vi "参数配置.vi"() -> ()   [LabVIEW 2012]
doc: "打开板卡操作，输出板卡句柄！当有多个板卡时，根据板卡索引号打开不同板卡！\n如果同时使用一块板卡的多种功能，可将输出句柄连接到不同的功能任务中。\n此VI是创建所有任务的前提！"
panel:
  in  "50_100HZ 2":u32(ring) items=["50Hz脉冲", "100Hz脉冲"]
  in  "50_100HZ":u32(ring) items=["50Hz脉冲", "100Hz脉冲"]
  in  "马尔科夫脉冲强度 2":u32(ring) items=["0dB", "3dB", "6dB", "9dB", "12dB", "15dB", "18dB"]
  in  "马尔科夫种类 2":u32(ring) items=["弱马尔科夫", "中马尔科夫", "强马尔科夫"]
  in  "脉冲噪声开关 2":bool=TRUE
  in  "工频异步脉冲强度 2":u32(ring) items=["0dB", "3dB", "6dB", "9dB", "12dB", "15dB", "18dB"]
  in  "脉冲种类 2":u32(ring) items=["50KHz脉冲", "100KHz脉冲", "200KHz脉冲"]
  in  "工频异步噪声开关 2":bool=TRUE
  in  "周期噪声强度 2":u32(ring) items=["0dB", "3dB", "6dB", "9dB", "12dB", "15dB", "18dB"]
  in  "工频同步噪声开关 2":bool=TRUE
  in  "窄带噪声强度 2":u32(ring) items=["0dB", "3dB", "6dB", "9dB", "12dB", "15dB"]
  in  "11MHz 2":bool
  in  "7MHz 2":bool
  in  "3MHz 2":bool=TRUE
  in  "窄带噪声开关 2":bool=TRUE
  in  "白噪声色噪声切换 2":bool=TRUE
  in  "背景噪声开关 2":bool=TRUE
  in  "背景噪声强度 2":u32(ring) items=["0dB", "3dB", "6dB", "9dB", "12dB", "15dB", "18dB"]
  out "Points to Date 3":u32 caption="当前点数"
  out "Number Unread 3":i32 caption="未读取数字"
  out "Buffer Size 3":i32 caption="缓冲区大小"
  in  "马尔科夫脉冲强度":u32(ring) items=["0dB", "3dB", "6dB", "9dB", "12dB", "15dB", "18dB"]
  in  "马尔科夫种类":u32(ring) items=["弱马尔科夫", "中马尔科夫", "强马尔科夫"]
  in  "脉冲噪声开关":bool=TRUE
  in  "工频异步脉冲强度":u32(ring) items=["0dB", "3dB", "6dB", "9dB", "12dB", "15dB", "18dB"]
  in  "脉冲种类":u32(ring) items=["50KHz脉冲", "100KHz脉冲", "200KHz脉冲"]
  in  "工频异步噪声开关":bool=TRUE
  in  "周期噪声强度":u32(ring) items=["0dB", "3dB", "6dB", "9dB", "12dB", "15dB", "18dB"]
  in  "工频同步噪声开关":bool=TRUE
  in  "窄带噪声强度":u32(ring) items=["0dB", "3dB", "6dB", "9dB", "12dB", "15dB"]
  in  "11MHz":bool
  in  "7MHz":bool
  in  "3MHz":bool=TRUE
  in  "窄带噪声开关":bool=TRUE
  in  "白噪声色噪声切换":bool=TRUE
  in  "背景噪声开关":bool=TRUE
  in  "背景噪声强度":u32(ring) items=["0dB", "3dB", "6dB", "9dB", "12dB", "15dB", "18dB"]
  in  "取消按钮":bool
  in  "后向信道参数选择":u16(ring)=1 items=["禁用信道", "接入参考信道  类型1", "接入参考信道  类型2", "接入参考信道  类型3", "接入参考信道  类型4", "接入参考信道  类型5", "室内信道 类型1", "室内信道 类型2", "室内信道 类型3", "室内信道 类型4", "来自配置文件"]
  in  "布尔 4":bool
  in  "后项配置文件路径":path
  in  "前向信道参数选择":u16(ring)=6 items=["禁用信道", "接入参考信道  类型1", "接入参考信道  类型2", "接入参考信道  类型3", "接入参考信道  类型4", "接入参考信道  类型5", "室内信道  类型1", "室内信道  类型2", "室内信道  类型3", "室内信道  类型4", "来自配置文件"]
  in  "布尔 3":bool
  in  "前向配置文件路径":path
  out "Points to Date":u32 caption="当前点数"
  out "Number Unread":i32 caption="未读取数字"
  out "Buffer Size":i32 caption="缓冲区大小"
  in  "确定按钮":bool
  # "按下“绘制”按钮时，通过打开的子VI显示最近获取的1024个数据点，然后进行绘制。"
  # "背景噪声"
  # "背景噪声"
  # "窄带噪声"
  # "窄带噪声"
  # "与工频同步的周期噪声"
  # "与工频同步的周期噪声"
  # "与工频异步的周期噪声"
  # "与工频异步的周期噪声"
  # "脉冲噪声"
  # "脉冲噪声"
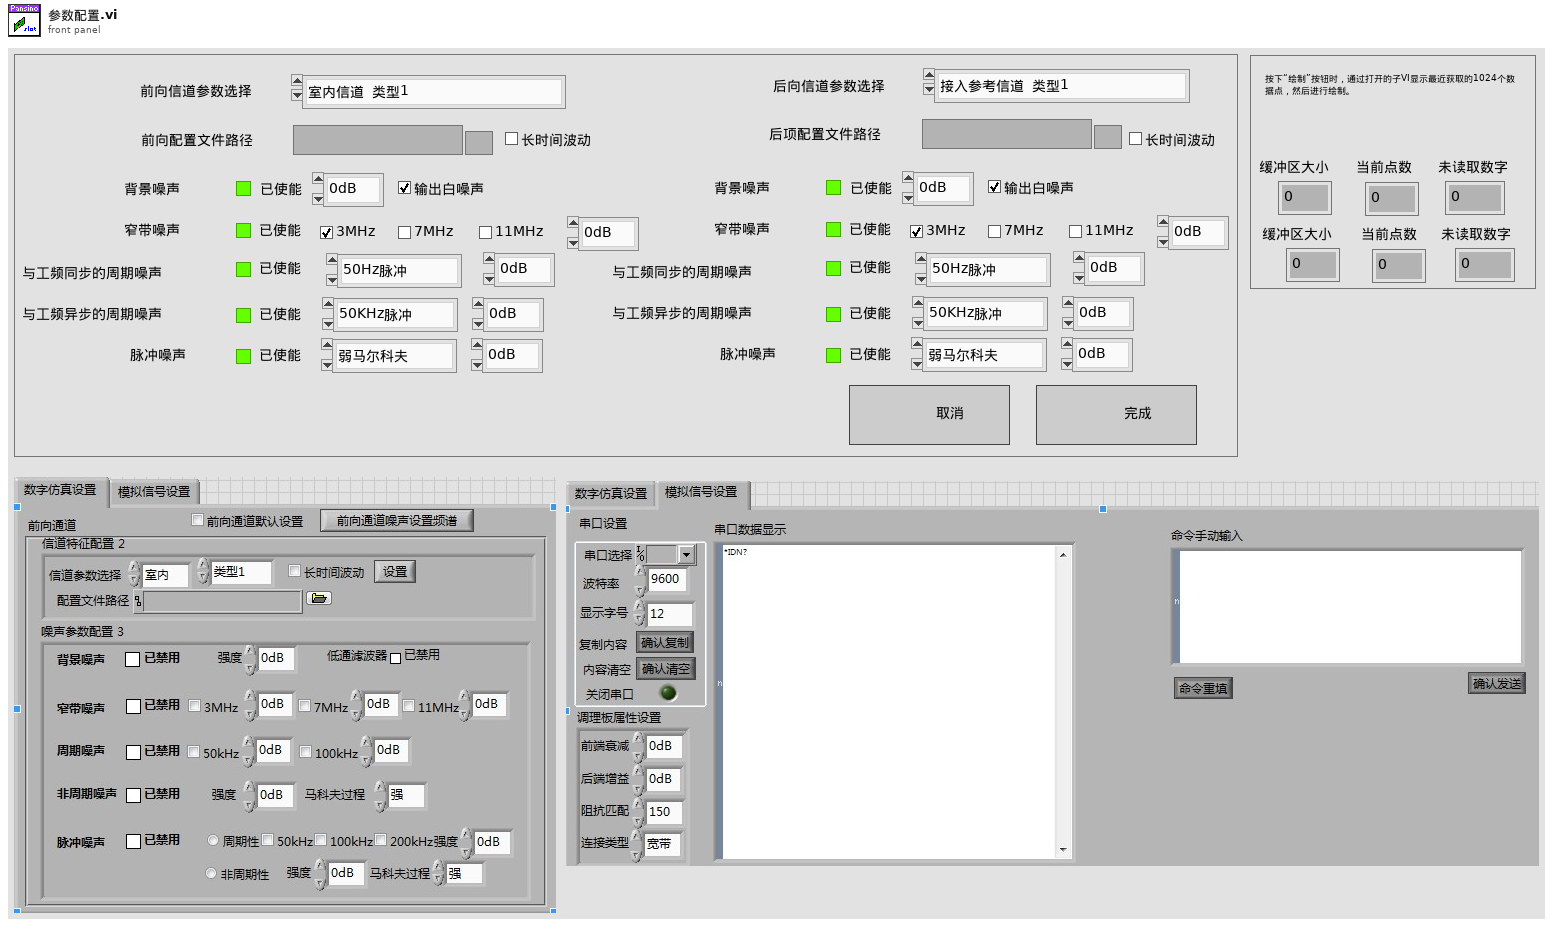
[diagram p1: front panel]
types:
  T1 = enum16{"empty", "write", "read oldest (queue)", "read newest (stack)", "read all"}
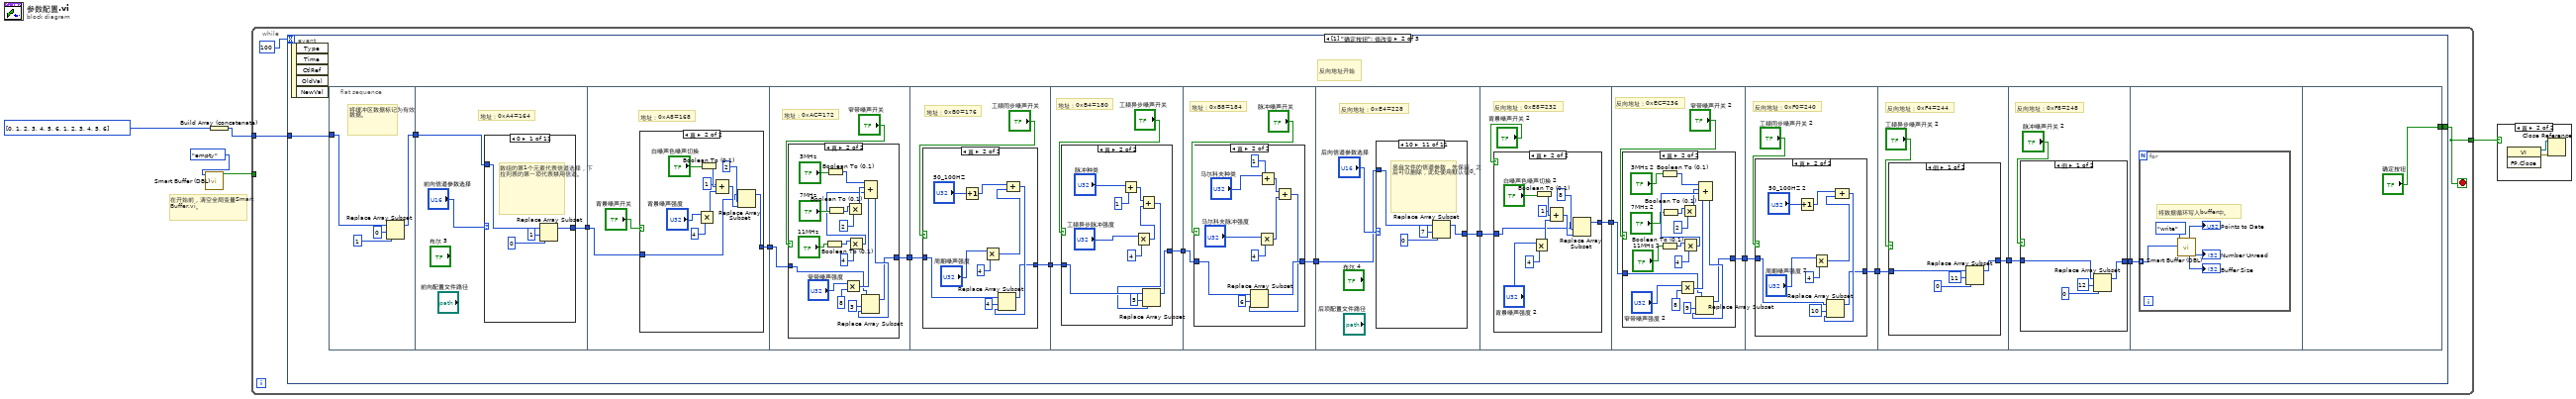
[diagram p0: block diagram]
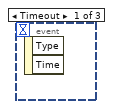
[diagram p3: hidden frame]
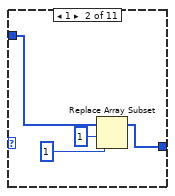
[diagram p4: hidden frame]
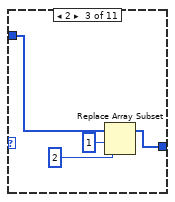
[diagram p5: hidden frame]
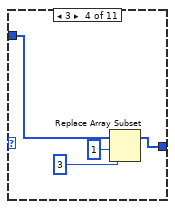
[diagram p6: hidden frame]
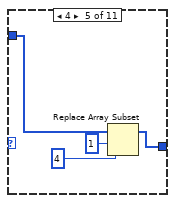
[diagram p7: hidden frame]
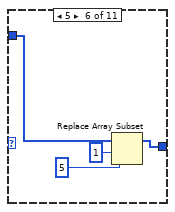
[diagram p8: hidden frame]
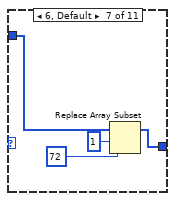
[diagram p9: hidden frame]
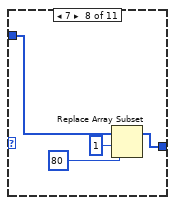
[diagram p10: hidden frame]
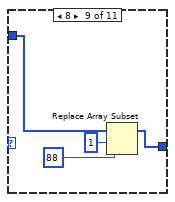
[diagram p11: hidden frame]
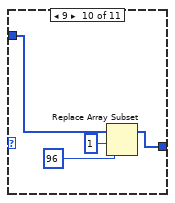
[diagram p12: hidden frame]
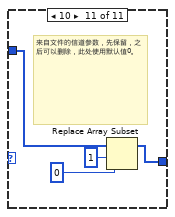
[diagram p13: hidden frame]
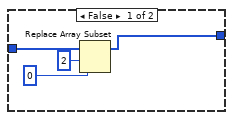
[diagram p14: hidden frame]
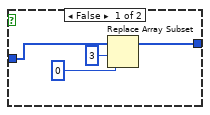
[diagram p15: hidden frame]
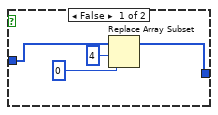
[diagram p16: hidden frame]
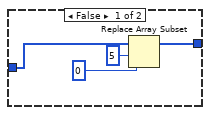
[diagram p17: hidden frame]
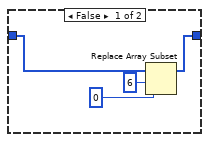
[diagram p18: hidden frame]
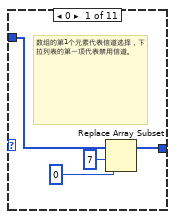
[diagram p19: hidden frame]
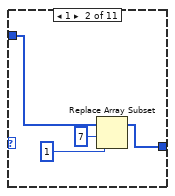
[diagram p20: hidden frame]
diagram:
  # "在开始前，清空全局变量Smart Buffer.vi。"
  n1 = call "Smart Buffer (DBL).vi"("mode"=T1."empty") -> ("output valid? [read]"=w4:bool)  [unwired: 5 in, 5 out]
  n2 = Build Array (concatenate)(i32[] [0, 1, 2, 3, 4, 5, 6, 1, 2, 3, 4, 5, 6] ("元素")) -> (w1:i32[])
  n3 = while {
    tunnel: w4 -> [_]
    tunnel: [w7] -> w3
    tunnel: w1 -> [w6]
    stop <- w7 stop-if-true
    n4 = event shown="[1] \"确定按钮\": 值改变" {
      selector: _ -> [_ _ _]
      dyn-events: _ -> [_ _ _]
      timeout: 100 -> [_ _ _]
      tunnel: [_ w16 "取消按钮"] -> w7
      tunnel: w6 -> [_ w23 w318]
      event Timeout {
        n5 = event-data() -> ()  [unwired: 1 in, 2 out]
      }
      event "确定按钮": Value Change {
        # "反向地址开始"
        n6 = event-data() -> ()  [unwired: 1 in, 5 out]
        n7 = flat-sequence {
          tunnel: w23 -> [w25]
          tunnel: [w24] -> w15
          tunnel: [w28] -> w22
          tunnel: w15 -> [w29]
          tunnel: w22 -> [w76]
          tunnel: [w75] -> w21
          tunnel: w21 -> [w93]
          tunnel: [w92] -> w20
          tunnel: w20 -> [w117]
          tunnel: [w116] -> w19
          tunnel: w19 -> [w133]
          tunnel: [w132] -> w18
          tunnel: w18 -> [w150]
          tunnel: [w149] -> w17
          tunnel: w17 -> [w167]
          tunnel: [w166] -> w13
          tunnel: w13 -> [w214]
          tunnel: [w213] -> w12
          tunnel: w12 -> [w231]
          tunnel: [w230] -> w11
          tunnel: w11 -> [w255]
          tunnel: [w254] -> w10
          tunnel: w10 -> [w272]
          tunnel: [w270] -> w9
          tunnel: [w287] -> w14
          tunnel: w9 -> [w288]
          tunnel: w14 -> [w304]
          tunnel: ["确定按钮"] -> w16
          frame #0 {
            # "将缓冲区数据标记为有效数据。"
            n8 = Replace Array Subset(array=w25, new element=1 ("新元素/子数组"), index=0 ("索引")) -> (w24:i32[])
          }
          frame #1 {
            # "地址：0xA4=164"
            n9 = case shown="0" "前向信道参数选择" {
              tunnel: w29 -> [w34 w36 w39 w44 w48 w51 w55 w59 w63 w67 w71]
              tunnel: [w31 w35 w40 w43 w47 w52 w56 w60 w64 w68 w72] -> w28
              frame 0 {
                # "数组的第1个元素代表信道选择，下拉列表的第一项代表禁用信道。"
                n10 = Replace Array Subset(array=w34, new element=0 ("新元素/子数组"), index=1 ("索引")) -> (w31:i32[])
              }
              frame 1 {
                n11 = Replace Array Subset(array=w36, new element=1 ("新元素/子数组"), index=1 ("索引")) -> (w35:i32[])
              }
              frame 2 {
                n12 = Replace Array Subset(array=w39, new element=2 ("新元素/子数组"), index=1 ("索引")) -> (w40:i32[])
              }
              frame 3 {
                n13 = Replace Array Subset(array=w44, new element=3 ("新元素/子数组"), index=1 ("索引")) -> (w43:i32[])
              }
              frame 4 {
                n14 = Replace Array Subset(array=w48, new element=4 ("新元素/子数组"), index=1 ("索引")) -> (w47:i32[])
              }
              frame 5 {
                n15 = Replace Array Subset(array=w51, new element=5 ("新元素/子数组"), index=1 ("索引")) -> (w52:i32[])
              }
              frame 6, Default {
                n16 = Replace Array Subset(array=w55, new element=72 ("新元素/子数组"), index=1 ("索引")) -> (w56:i32[])
              }
              frame 7 {
                n17 = Replace Array Subset(array=w59, new element=80 ("新元素/子数组"), index=1 ("索引")) -> (w60:i32[])
              }
              frame 8 {
                n18 = Replace Array Subset(array=w63, new element=88 ("新元素/子数组"), index=1 ("索引")) -> (w64:i32[])
              }
              frame 9 {
                n19 = Replace Array Subset(array=w67, new element=96 ("新元素/子数组"), index=1 ("索引")) -> (w68:i32[])
              }
              frame 10 {
                # "来自文件的信道参数，先保留，之后可以删除，此处使用默认值0。"
                n20 = Replace Array Subset(array=w71, new element=0 ("新元素/子数组"), index=1 ("索引")) -> (w72:i32[])
              }
            }
          }
          frame #2 {
            # "地址：0xA8=168"
            n21 = case shown="真" "背景噪声开关" {
              tunnel: w76 -> [w79 w83]
              tunnel: [w78 w84] -> w75
              frame False {
                n22 = Replace Array Subset(array=w79, new element=0 ("新元素/子数组"), index=2 ("索引")) -> (w78:i32[])
              }
              frame True {
                n23 = Multiply(x="背景噪声强度", y=u32 4) -> (x*y=w87:u32)
                n24 = Boolean To (0,1)(Boolean="白噪声色噪声切换") -> (0, 1=w88:i16)
                n25 = Compound Arithmetic op=ADD(i16 1 ("值"), w88, w87) -> (w85:u32)
                n26 = Replace Array Subset(array=w83, new element=w85, index=2 ("索引")) -> (w84:i32[])
              }
            }
          }
          frame #3 {
            # "地址：0xAC=172"
            n27 = case shown="真" "窄带噪声开关" {
              tunnel: w93 -> [w96 w101]
              tunnel: [w95 w99] -> w92
              frame False {
                n28 = Replace Array Subset(array=w96, new element=0 ("新元素/子数组"), index=3 ("索引")) -> (w95:i32[])
              }
              frame True {
                n29 = Boolean To (0,1)(Boolean="11MHz") -> (0, 1=w110:i16)
                n30 = Boolean To (0,1)(Boolean="3MHz") -> (0, 1=w108:i16)
                n31 = Boolean To (0,1)(Boolean="7MHz") -> (0, 1=w109:i16)
                n32 = Multiply(x="窄带噪声强度", y=u32 8) -> (x*y=w104:u32)
                n33 = Multiply(x=w109, y=u32 2) -> (x*y=w107:u32)
                n34 = Multiply(x=w110, y=u32 4) -> (x*y=w106:u32)
                n35 = Compound Arithmetic op=ADD(w108, w107, w106, w104) -> (w100:u32)
                n36 = Replace Array Subset(array=w101, new element=w100, index=3 ("索引")) -> (w99:i32[])
              }
            }
          }
          frame #4 {
            # "地址：0xB0=176"
            n37 = case shown="真" "工频同步噪声开关" {
              tunnel: w117 -> [w120 w127]
              tunnel: [w119 w125] -> w116
              frame False {
                n38 = Replace Array Subset(array=w120, new element=0 ("新元素/子数组"), index=4 ("索引")) -> (w119:i32[])
              }
              frame True {
                n39 = Increment(x="50_100HZ") -> (x+1=w123:u32)
                n40 = Multiply(x="周期噪声强度", y=u32 4) -> (x*y=w129:u32)
                n41 = Compound Arithmetic op=ADD(w123, w129) -> (w126:u32)
                n42 = Replace Array Subset(array=w127, new element=w126, index=4 ("索引")) -> (w125:i32[])
              }
            }
          }
          frame #5 {
            # "地址：0xB4=180"
            n43 = case shown="真" "工频异步噪声开关" {
              tunnel: w133 -> [w136 w147]
              tunnel: [w135 w146] -> w132
              frame False {
                n44 = Replace Array Subset(array=w136, new element=0 ("新元素/子数组"), index=5 ("索引")) -> (w135:i32[])
              }
              frame True {
                n45 = Add(x="脉冲种类", y=u32 1) -> (x+y=w141:u32)
                n46 = Multiply(x="工频异步脉冲强度", y=u32 4) -> (x*y=w140:u32)
                n47 = Add(x=w141, y=w140) -> (x+y=w139:u32)
                n48 = Replace Array Subset(array=w147, new element=w139, index=5 ("索引")) -> (w146:i32[])
              }
            }
          }
          frame #6 {
            # "地址：0xB8=184"
            n49 = case shown="真" "脉冲噪声开关" {
              tunnel: w150 -> [w153 w164]
              tunnel: [w152 w163] -> w149
              frame False {
                n50 = Replace Array Subset(array=w153, new element=0 ("新元素/子数组"), index=6 ("索引")) -> (w152:i32[])
              }
              frame True {
                n51 = Multiply(x="马尔科夫脉冲强度", y=u32 4) -> (x*y=w157:u32)
                n52 = Add(x="马尔科夫种类", y=u32 1) -> (x+y=w162:u32)
                n53 = Add(x=w162, y=w157) -> (x+y=w156:u32)
                n54 = Replace Array Subset(array=w164, new element=w156, index=6 ("索引")) -> (w163:i32[])
              }
            }
          }
          frame #7 {
            # "反向地址：0xE4=228"
            n55 = case shown="10" "后向信道参数选择" {
              tunnel: w167 -> [w172 w174 w177 w182 w186 w189 w193 w197 w201 w205 w209]
              tunnel: [w169 w173 w178 w181 w185 w190 w194 w198 w202 w206 w210] -> w166
              frame 0 {
                # "数组的第1个元素代表信道选择，下拉列表的第一项代表禁用信道。"
                n56 = Replace Array Subset(array=w172, new element=0 ("新元素/子数组"), index=7 ("索引")) -> (w169:i32[])
              }
              frame 1 {
                n57 = Replace Array Subset(array=w174, new element=1 ("新元素/子数组"), index=7 ("索引")) -> (w173:i32[])
              }
              frame 2 {
                n58 = Replace Array Subset(array=w177, new element=2 ("新元素/子数组"), index=7 ("索引")) -> (w178:i32[])
              }
              frame 3 {
                n59 = Replace Array Subset(array=w182, new element=3 ("新元素/子数组"), index=7 ("索引")) -> (w181:i32[])
              }
              frame 4 {
                n60 = Replace Array Subset(array=w186, new element=4 ("新元素/子数组"), index=7 ("索引")) -> (w185:i32[])
              }
              frame 5 {
                n61 = Replace Array Subset(array=w189, new element=5 ("新元素/子数组"), index=7 ("索引")) -> (w190:i32[])
              }
              frame 6, Default {
                n62 = Replace Array Subset(array=w193, new element=72 ("新元素/子数组"), index=7 ("索引")) -> (w194:i32[])
              }
              frame 7 {
                n63 = Replace Array Subset(array=w197, new element=80 ("新元素/子数组"), index=7 ("索引")) -> (w198:i32[])
              }
              frame 8 {
                n64 = Replace Array Subset(array=w201, new element=88 ("新元素/子数组"), index=7 ("索引")) -> (w202:i32[])
              }
              frame 9 {
                n65 = Replace Array Subset(array=w205, new element=96 ("新元素/子数组"), index=7 ("索引")) -> (w206:i32[])
              }
              frame 10 {
                # "来自文件的信道参数，先保留，之后可以删除，此处使用默认值0。"
                n66 = Replace Array Subset(array=w209, new element=0 ("新元素/子数组"), index=7 ("索引")) -> (w210:i32[])
              }
            }
          }
          frame #8 {
            # "反向地址：0xE8=232"
            n67 = case shown="真" "背景噪声开关 2" {
              tunnel: w214 -> [w217 w222]
              tunnel: [w216 w221] -> w213
              frame False {
                n68 = Replace Array Subset(array=w217, new element=0 ("新元素/子数组"), index=8 ("索引")) -> (w216:i32[])
              }
              frame True {
                n69 = Multiply(x="背景噪声强度 2", y=u32 4) -> (x*y=w227:u32)
                n70 = Boolean To (0,1)(Boolean="白噪声色噪声切换 2") -> (0, 1=w226:i16)
                n71 = Compound Arithmetic op=ADD(i16 1 ("值"), w226, w227) -> (w229:u32)
                n72 = Replace Array Subset(array=w222, new element=w229, index=8 ("索引")) -> (w221:i32[])
              }
            }
          }
          frame #9 {
            # "反向地址：0xEC=236"
            n73 = case shown="真" "窄带噪声开关 2" {
              tunnel: w231 -> [w234 w239]
              tunnel: [w233 w238] -> w230
              frame False {
                n74 = Replace Array Subset(array=w234, new element=0 ("新元素/子数组"), index=9 ("索引")) -> (w233:i32[])
              }
              frame True {
                n75 = Boolean To (0,1)(Boolean="11MHz 2") -> (0, 1=w245:i16)
                n76 = Boolean To (0,1)(Boolean="3MHz 2") -> (0, 1=w247:i16)
                n77 = Boolean To (0,1)(Boolean="7MHz 2") -> (0, 1=w246:i16)
                n78 = Multiply(x="窄带噪声强度 2", y=u32 8) -> (x*y=w250:u32)
                n79 = Multiply(x=w246, y=u32 2) -> (x*y=w248:u32)
                n80 = Multiply(x=w245, y=u32 4) -> (x*y=w249:u32)
                n81 = Compound Arithmetic op=ADD(w247, w248, w249, w250) -> (w253:u32)
                n82 = Replace Array Subset(array=w239, new element=w253, index=9 ("索引")) -> (w238:i32[])
              }
            }
          }
          frame #10 {
            # "反向地址：0xF0=240"
            n83 = case shown="真" "工频同步噪声开关 2" {
              tunnel: w255 -> [w258 w264]
              tunnel: [w257 w263] -> w254
              frame False {
                n84 = Replace Array Subset(array=w258, new element=0 ("新元素/子数组"), index=10 ("索引")) -> (w257:i32[])
              }
              frame True {
                n85 = Increment(x="50_100HZ 2") -> (x+1=w261:u32)
                n86 = Multiply(x="周期噪声强度 2", y=u32 4) -> (x*y=w267:u32)
                n87 = Compound Arithmetic op=ADD(w261, w267) -> (w269:u32)
                n88 = Replace Array Subset(array=w264, new element=w269, index=10 ("索引")) -> (w263:i32[])
              }
            }
          }
          frame #11 {
            # "反向地址：0xF4=244"
            n89 = case shown="假" "工频异步噪声开关 2" {
              tunnel: w272 -> [w273 w278]
              tunnel: [w274 w277] -> w270
              frame False {
                n90 = Replace Array Subset(array=w273, new element=0 ("新元素/子数组"), index=11 ("索引")) -> (w274:i32[])
              }
              frame True {
                n91 = Add(x="脉冲种类 2", y=u32 1) -> (x+y=w284:u32)
                n92 = Multiply(x="工频异步脉冲强度 2", y=u32 4) -> (x*y=w285:u32)
                n93 = Add(x=w284, y=w285) -> (x+y=w286:u32)
                n94 = Replace Array Subset(array=w278, new element=w286, index=11 ("索引")) -> (w277:i32[])
              }
            }
          }
          frame #12 {
            # "反向地址：0xF8=248"
            n95 = case shown="假" "脉冲噪声开关 2" {
              tunnel: w288 -> [w290 w295]
              tunnel: [w291 w294] -> w287
              frame False {
                n96 = Replace Array Subset(array=w290, new element=0 ("新元素/子数组"), index=12 ("索引")) -> (w291:i32[])
              }
              frame True {
                n97 = Multiply(x="马尔科夫脉冲强度 2", y=u32 4) -> (x*y=w303:u32)
                n98 = Add(x="马尔科夫种类 2", y=u32 1) -> (x+y=w301:u32)
                n99 = Add(x=w301, y=w303) -> (x+y=w296:u32)
                n100 = Replace Array Subset(array=w295, new element=w296, index=12 ("索引")) -> (w294:i32[])
              }
            }
          }
          frame #13 {
            n101 = for {
              tunnel: w304 -> [w305] mode=indexing
              # "将数据循环写入buffer中。"
              n102 = call "Smart Buffer (DBL).vi"("new element [write]"=w305, "mode"=T1."write") -> ("number unread after"=→"Number Unread":i32, "buffer size"=→"Buffer Size":i32, "number written after"=→"Points to Date":u32)  [unwired: 4 in, 3 out]
            }
          }
          frame #14 {
          }
        }
      }
      event "取消按钮": Value Change {
        # "将数据循环写入buffer中,此处只写入了一个0，故buffer中只有一个元素0。"
        # "将缓冲区数据标记为有效数据。"
        n103 = event-data() -> ()  [unwired: 1 in, 5 out]
        n104 = Replace Array Subset(array=w318, new element=0 ("新元素/子数组"), index=0 ("索引")) -> (w317:i32[])
        n105 = Index Array(array=w317, index=0 ("索引")) -> (element=w311:i32)
        n106 = call "Smart Buffer (DBL).vi"("new element [write]"=w311, "mode"=T1."write") -> ("number unread after"=→"Number Unread 3":i32, "buffer size"=→"Buffer Size 3":i32, "number written after"=→"Points to Date 3":u32)  [unwired: 4 in, 3 out]
      }
    }
  }
  n107 = case shown="真" w3 {
    frame False {
    }
    frame True {
      n108 = invoke class="VI" method="FP.Close"() -> (reference out=w322:refnum<vi>, error out=w323:errorcluster)  [unwired: 3 in, 1 out]
      n109 = Close Reference(reference=w322, error in (no error)=w323) -> ()  [unwired: 1 out]
    }
  }
